vi "unused_getType.vi"(8 "error in (no error)":errorcluster, 11 "GObject in":refnum<class "GObject.lvclass">) -> (0 "error out":errorcluster, 2 "type":refnum<vi>, 3 "GObject out":refnum<class "GObject.lvclass">)   [LabVIEW 2023]
uses:
  GObject.lvclass/GObject.ctl
  GObject.lvclass
  C:/projects/TLC_Scripto/Source/Generic/Generic.lvclass
  C:/projects/TLC_Scripto/Source/GObject/GObject.lvclass
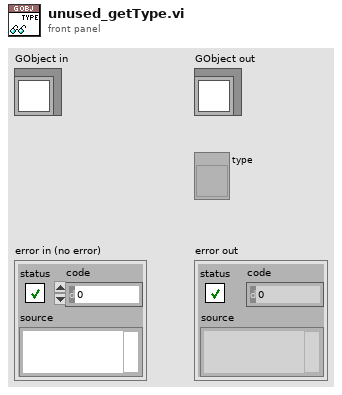
[diagram p1: front panel]
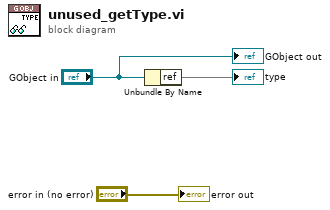
[diagram p0: block diagram]
diagram:
  n1 = Unbundle By Name("GObject in") -> ("ref"=→"type")
  "error out" <- "error in (no error)"
  "GObject out" <- "GObject in"
